vi "TDT-Endpoint To Sequential Connection Number.vi"(0 "Device":T1, 2 "Section":string, 9 "Endpoints":string[](array[string]), 11 "error in (no error)":errorcluster) -> (8 "SeqCxnNum":i32[](array[numeric]), 15 "error out":errorcluster)   [LabVIEW 2020]
uses:
  Typedefs/TDT-Device ID.ctl
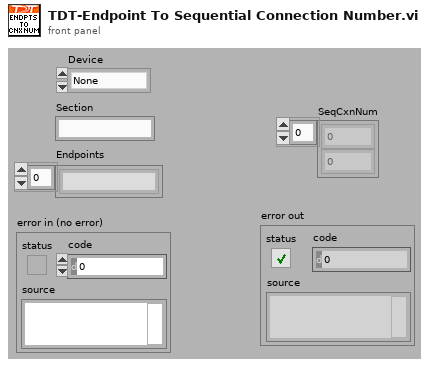
[diagram p1: front panel]
types:
  T1 = typedef "TDT-Device ID.ctl" = enum16{"None", "PA5", "RP2", "RL2", "RA16", "RV8", "RX5", "RX6", "RX7", "RX8", "RZ2", "RZ5", "RZ6"}
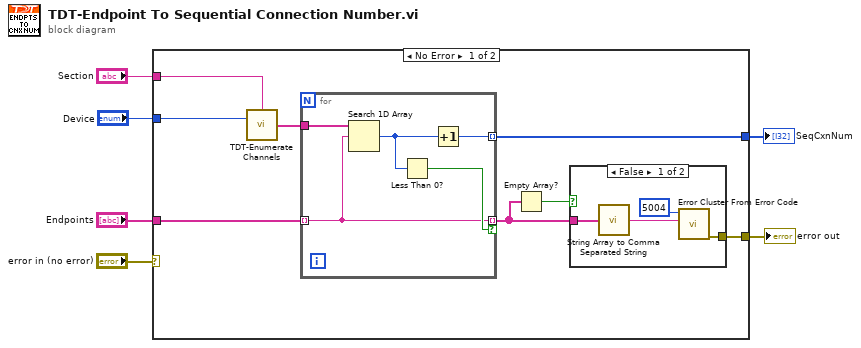
[diagram p0: block diagram]
diagram:
  n1 = case shown="No Error" "error in (no error)" {
    selector: "error in (no error)" -> [_ w24]
    tunnel: [w13 _] -> w6
    tunnel: [w12 w24] -> w5
    tunnel: "Section" -> [w11 _]
    tunnel: "Endpoints" -> [w8 _]
    tunnel: "Device" -> [w7 _]
    frame No Error {
      n2 = call "TDT-Enumerate Channels.vi"("Type"=w11, "IO Device"=w7) -> ("IO Channels"=w14:string[])  [unwired: 13 in]
      n3 = for {
        tunnel: w14 -> [w19]
        tunnel: [w16] -> w13 mode=indexing
        tunnel: [w15] -> w10 mode=indexing if=w17
        tunnel: w8 -> [w15] mode=indexing
        n4 = Search 1D Array(1D array=w19, element=w15) -> (index of element=w18:i32)  [unwired: 1 in]
        n5 = Less Than 0?(x=w18) -> (x < 0?=w17:bool)
        n6 = Increment(x=w18) -> (x+1=w16:i32)
      }
      n7 = Empty Array?(array=w10) -> (empty?=w9:bool)
      n8 = case shown="False" w9 {
        tunnel: [w23 _] -> w12
        tunnel: w10 -> [w21 _]
        frame False {
          n9 = call "String Array to Comma Separated String.vi"("String Array"=w21) -> ("comma separated string"=w20:string)
          n10 = call <vilib>:"Error Cluster From Error Code.vi"("error message (\"\")"=w20, "error code (0)"=5004) -> ("error out"=w23:errorcluster)  [unwired: 7 in]
        }
        frame True {
        }
      }
    }
    frame Error {
    }
  }
  "error out" <- w5
  "SeqCxnNum" <- w6
